vi "AMPM Configure.vi"(0 "RFmx Handle In":refnum<k21>, 1 "Selector String":string, 5 "RFmx SpecAn AMPM Configuration":T1={"Measurement Interval (s)"=0.0001, "DUT Input Power (dBm)"=-20.0, "Signal Type"=0, "Reference Waveform"={"Waveform Name"="Wfm", "Waveform"={"x0"=0.0, "dx"=0.0, "y"=[]}, "Signal Bandwidth (Hz)"=0.0, "PAPR (dB)"=0.0, "Burst Length (s)"=0.0, "Sample Rate"=0.0, "Burst Start Locations"=[], "Burst Stop Locations"=[], "Idle Duration Present?"=FALSE, "Runtime Scaling"=0.0}} {"Reference Waveform"."Runtime Scaling" format="%#_6p"; "Reference Waveform"."Sample Rate" format="%#_6p"; "Reference Waveform"."Burst Length (s)" format="%#_6p"; "Reference Waveform"."PAPR (dB)" format="%.2f"; "Reference Waveform"."Signal Bandwidth (Hz)" format="%#_6p"; "Reference Waveform"."Waveform"."y" format="%.2f"; "Reference Waveform"."Waveform"."dx" format="%^.2e"; "Reference Waveform"."Waveform"."x0" format="%^.2e"; "Signal Type" items=["Modulated", "Tones"]; "DUT Input Power (dBm)" format="%.2p"; "Measurement Interval (s)" format="%.2p"}, 11 "error in (no error)":errorcluster) -> (4 "RFmx Handle Out":refnum<k21>, 15 "error out":errorcluster)   [LabVIEW 2016, in "RFmxSpecAn.lvlib"]
uses:
  RFmxSpecAn.lvlib
  Typedefs/AMPM Configuration.ctl
  SG/Typedefs/Waveform.ctl
  <resource>/objmgr/RFmxSpecAn.rc
  SG/SG.lvlib
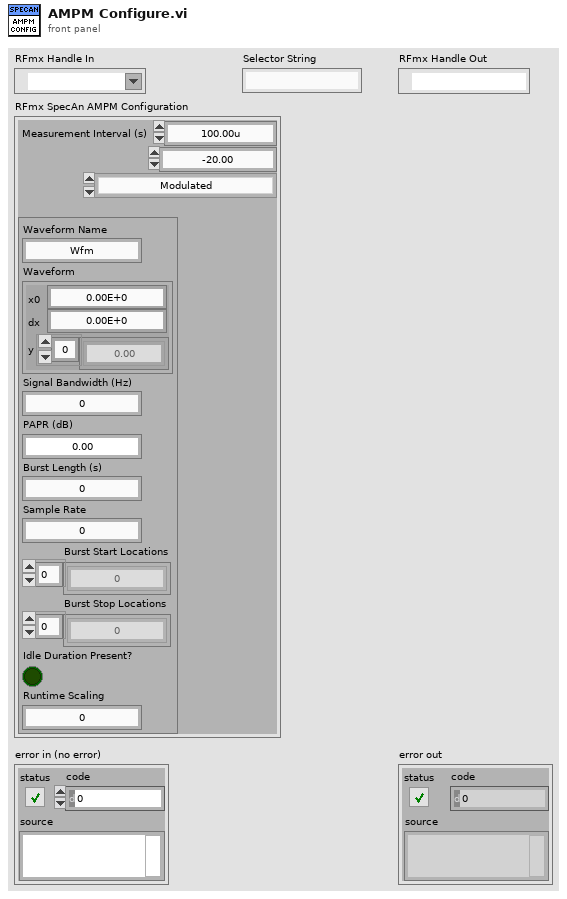
[diagram p1: front panel]
types:
  T1 = typedef "RFmxSpecAn.lvlib/AMPM Configuration.ctl" = cluster{"Measurement Interval (s)":dbl, "DUT Input Power (dBm)":dbl, "Signal Type":i32, "Reference Waveform":T2}
  T2 = typedef "SG.lvlib/Waveform.ctl" = cluster{"Waveform Name":string, "Waveform":cluster{"x0":dbl, "dx":dbl, "y":csg[]}, "Signal Bandwidth (Hz)":dbl, "PAPR (dB)":dbl, "Burst Length (s)":dbl, "Sample Rate":dbl, "Burst Start Locations":i32[], "Burst Stop Locations":i32[], "Idle Duration Present?":bool, "Runtime Scaling":dbl}
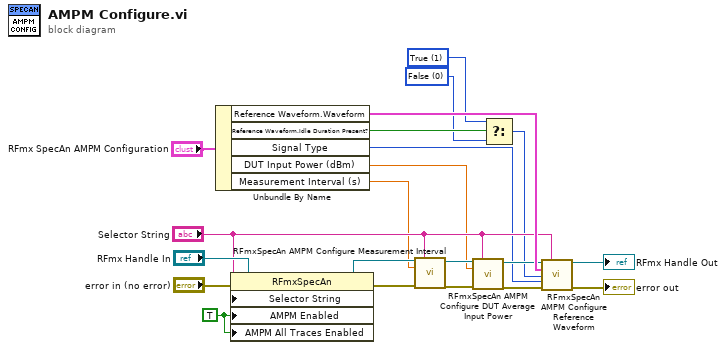
[diagram p0: block diagram]
diagram:
  w3 = 0 items=["False", "True"] ("Idle Duration Present")
  w6 = 1 items=["False", "True"] ("Idle Duration Present")
  w8 = TRUE ("AMPM Enabled")
  n1 = Unbundle By Name("RFmx SpecAn AMPM Configuration") -> ("Reference Waveform.Waveform"=w20:cluster{"x0":dbl, "dx":dbl, "y":csg[]}, "Reference Waveform.Idle Duration Present?"=w4:bool, "Signal Type"=w7:i32, "DUT Input Power (dBm)"=w2:dbl, "Measurement Interval (s)"=w1:dbl)
  n2 = property class="RFmxSpecAn"(reference="RFmx Handle In", error in="error in (no error)", "Selector String"="Selector String", "AMPM Enabled"=w8, "AMPM All Traces Enabled"=w8) -> (reference out=w12:refnum<k21>, error out=w10:errorcluster)
  n3 = call <vilib>:"RFmxSpecAn AMPM Configure Measurement Interval.vi"("Instrument Handle In"=w12, "Selector String"="Selector String", "Measurement Interval (s)"=w1, "error in (no error)"=w10) -> ("Instrument Handle Out"=w19:refnum<k21>, "error out"=w18:errorcluster)  [unwired: 10 in]
  n4 = call <vilib>:"RFmxSpecAn AMPM Configure DUT Average Input Power.vi"("Instrument Handle In"=w19, "Selector String"="Selector String", "DUT Average Input Power (dBm)"=w2, "error in (no error)"=w18) -> ("Instrument Handle Out"=w17:refnum<k21>, "error out"=w16:errorcluster)  [unwired: 10 in]
  n5 = Select(t=w6, s=w4, f=w3) -> (s? t:f=w5:i32)
  n6 = call <vilib>:"RFmxSpecAn AMPM Configure Reference Waveform.vi"("Instrument Handle In"=w17, "Selector String"="Selector String", "Reference Waveform"=w20, "Idle Duration Present"=w5, "Signal Type"=w7, "error in (no error)"=w16) -> ("Instrument Handle Out"=→"RFmx Handle Out":refnum<k21>, "error out"=→"error out":errorcluster)  [unwired: 8 in]
